vi "set_config_cluster.vi"(8 "error in (no error)":errorcluster, 10 "config cluster variant":variant, 11 "SweepDL090926Automation in":refnum<class "SweepDL090926Automation.lvclass">) -> (0 "error out":errorcluster, 3 "SweepDL090926Automation out":refnum<class "SweepDL090926Automation.lvclass">)   [LabVIEW 2010, in "SweepDL090926Automation.lvclass"]
uses:
  SweepDL090926Automation.lvclass
  SweepDL090926Automation.lvclass/SweepDL090926Automation.ctl
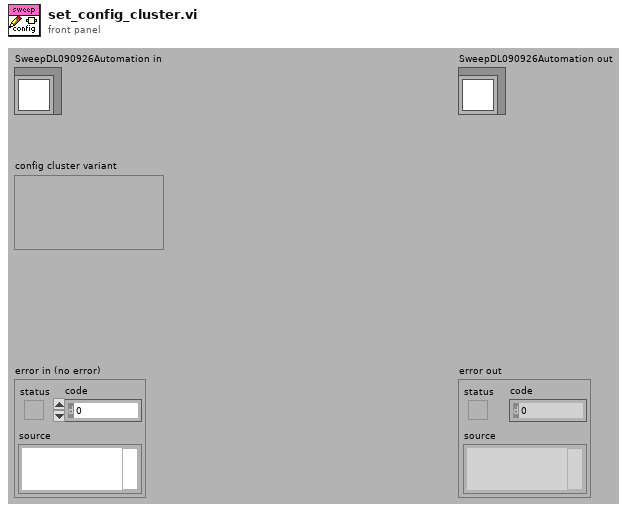
[diagram p1: front panel]
types:
  T1 = typedef "SweepDL090926Automation.lvclass/config_data_cluster.ctl" = cluster{"imaging-mode sequence":T2[]}
  T2 = typedef "plugin_specification.ctl" = cluster{"class path":string, "configuration":string, "label":string, "settings name":string}
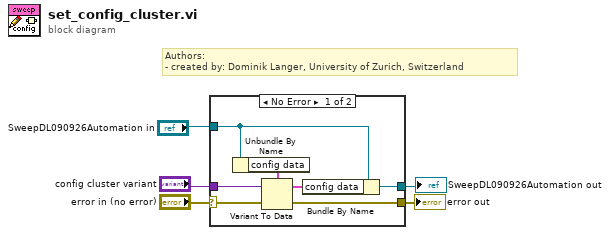
[diagram p0: block diagram]
diagram:
  # "Authors: \n- created by: Dominik Langer, University of Zurich, Switzerland"
  n1 = case shown="No Error" "error in (no error)" {
    selector: "error in (no error)" -> [w10 w13]
    tunnel: "SweepDL090926Automation in" -> [w8 w14]
    tunnel: [w7 w13] -> w1
    tunnel: [w6 w14] -> w2
    tunnel: "config cluster variant" -> [w9 _]
    frame No Error {
      n2 = Unbundle By Name(w8) -> ("config data"=w12:T1)
      n3 = Variant To Data(error in=w10, Variant=w9, type=w12) -> (error out=w7:errorcluster, data=w11:T1)
      n4 = Bundle By Name(cluster=w8, "config data"=w11) -> (w6:refnum<class "SweepDL090926Automation.lvclass">)
    }
    frame Error {
    }
  }
  "error out" <- w1
  "SweepDL090926Automation out" <- w2
